vi "AB_820_850_Project_SourceItems.vi"(5 "Provider Item":T1, 7 "action":T3, 8 "error in (no error)":errorcluster, 9 "buildType":T2, 10 "oldBuildObject":T1, 11 "buildObject":T1) -> (0 "error out":errorcluster, 3 "buildObject out":T1, 4 "usedDestinations":i32[](array[numeric]))   [LabVIEW 2020]
doc: "Reads and writes the data to the object property bag."
uses:
  <resource>/Framework/Providers/API/ItemRef.ctl
  <vilib>/AppBuilder/RW_Project/AB_RW_Project_PropBag_ArrayAction.ctl
  <vilib>/AppBuilder/AB_BuildType.ctl
  <vilib>/AppBuilder/RW_Project/AB_RW_Project_Source_Data_for_Previous.ctl
  <vilib>/Utility/lvfile.llb/LVFileType.ctl
  <vilib>/AppBuilder/RW_Project/AB_RW_Project_PropBag_Action.ctl
  <vilib>/AppBuilder/AB_Source_Inclusion.ctl
  <vilib>/Utility/lvfile.llb/NI_FileType.lvlib
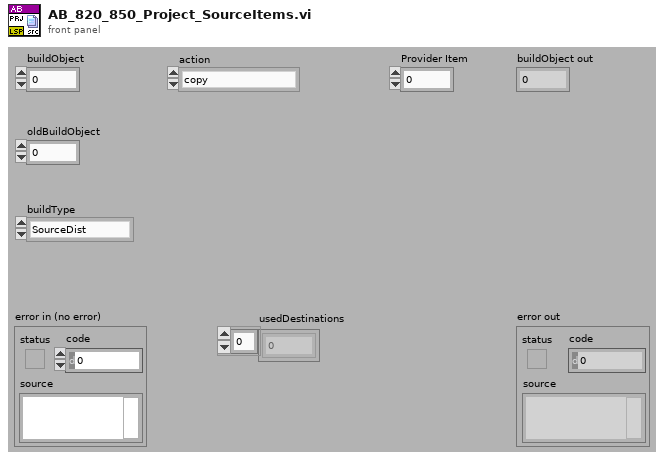
[diagram p1: front panel]
types:
  T1 = typedef "ItemRef.ctl" = u64
  T2 = typedef "AB_BuildType.ctl" = enum16{"SourceDist", "EXE", "DLL", "RTExe"}
  T3 = typedef "AB_RW_Project_PropBag_ArrayAction.ctl" = enum16{"copy", "saveForPrevious", "loadFromPrevious", "clear"}
  T4 = typedef "AB_RW_Project_Source_Data_for_Previous.ctl" = cluster{"buildType":T2, "folder":bool, "linkerInfo":cluster{"path":path, "delimited name":string, "type":T5, "iState":u32, "iStyle":u16, "wStyle":u16, "buttons":u16, "viflags":u32, "viflags2":u32, "links":u32[]}, "isLibrary":bool}
  T5 = typedef "NI_FileType.lvlib/LVFileType.ctl" = enum32{"Invalid file", "Unknown type", "Instrument", "Control", "Polymorphic VI", "Project", "Library", "LVClass", "XControl", "XNode", "Shared library", ".NET assembly", "ActiveX interface", "CIN", "Run-time menu", "Palette menu", "Help file", "LLB", "XNode Edit Dependency", "Class Private Data Control", "Statechart", "MathScript .m file", "Ladder Diagram", "LVLibp", "XNode Build Dependency"}
  T6 = typedef "AB_RW_Project_PropBag_Action.ctl" = enum16{"read", "write", "clear", "readPrevious", "writePrevious", "clearPrevious"}
  T7 = typedef "AB_Source_Inclusion.ctl" = enum16{"IncludeIfReferenced", "Include", "Exclude", "TopLevel"}
  T8 = cluster{"itemID":string, "sourceInclusion":T7, "destinationIndex":i32, "properties":cluster{"sourcePropertyType":enum16{"Remove block diagram", "Remove front panel", "Password", "Window has title bar", "Show menu bar", "Show vertical scroll bar", "Show horizontal scroll bar", "Show toolbar", "Show Abort button", "Show fp when called", "Window behavior", "Allow user to close window", "Window run-time position", "Run when opened", "Allow debugging", "Auto error handling"}, "value":variant}[], "newName":string, "lvfile":bool}
  T9 = cluster{"LLBtopLevel":bool, "privateDataControl":bool}
  T10 = typedef "ABAPI Dist VI Proto Info.ctl" = cluster{"cptm":string, "params":cluster{"name":string, "dir":enum32{"in", "out", "in/out", "length"}, "inputIdx":i32, "outputIdx":i32, "passBy":i32, "lenInput":i32, "lenOutput":i32}[], "callingConv":i32, "name":string}
  T11 = cluster{"applyInclusion":bool, "applyDestination":bool, "applyProperties":bool, "applyPassword":bool, "applyPrefix":bool, "applySaveSetttings":bool}
  T12 = cluster{"relinkCallers":bool, "atomicCopy":bool, "allowMissingMembers":bool}
  T13 = cluster{"Source":cluster{"itemID":string, "sourceInclusion":T7, "destinationIndex":i32, "properties":cluster{"sourcePropertyType":enum16{"Remove block diagram", "Remove front panel", "Password", "Window has title bar", "Show menu bar", "Show vertical scroll bar", "Show horizontal scroll bar", "Show toolbar", "Show Abort button", "Show fp when called", "Window behavior", "Allow user to close window", "Window run-time position", "Run when opened", "Allow debugging", "Auto error handling"}, "value":variant}[], "newName":string, "lvfile":bool}, "Container":cluster{"applyInclusion":bool, "applyDestination":bool, "applyProperties":bool, "applyPassword":bool, "applyPrefix":bool, "applySaveSetttings":bool}}
  T14 = cluster{"path":path, "delimited name":string, "type":T5, "iState":u32, "iStyle":u16, "wStyle":u16, "buttons":u16, "viflags":u32, "viflags2":u32, "links":u32[]}
  T15 = cluster{"dataSource out":cluster{"itemID":string, "sourceInclusion":T7, "destinationIndex":i32, "properties":cluster{"sourcePropertyType":enum16{"Remove block diagram", "Remove front panel", "Password", "Window has title bar", "Show menu bar", "Show vertical scroll bar", "Show horizontal scroll bar", "Show toolbar", "Show Abort button", "Show fp when called", "Window behavior", "Allow user to close window", "Window run-time position", "Run when opened", "Allow debugging", "Auto error handling"}, "value":variant}[], "newName":string, "lvfile":bool}, "dataSource out":cluster{"applyInclusion":bool, "applyDestination":bool, "applyProperties":bool, "applyPassword":bool, "applyPrefix":bool, "applySaveSetttings":bool}}
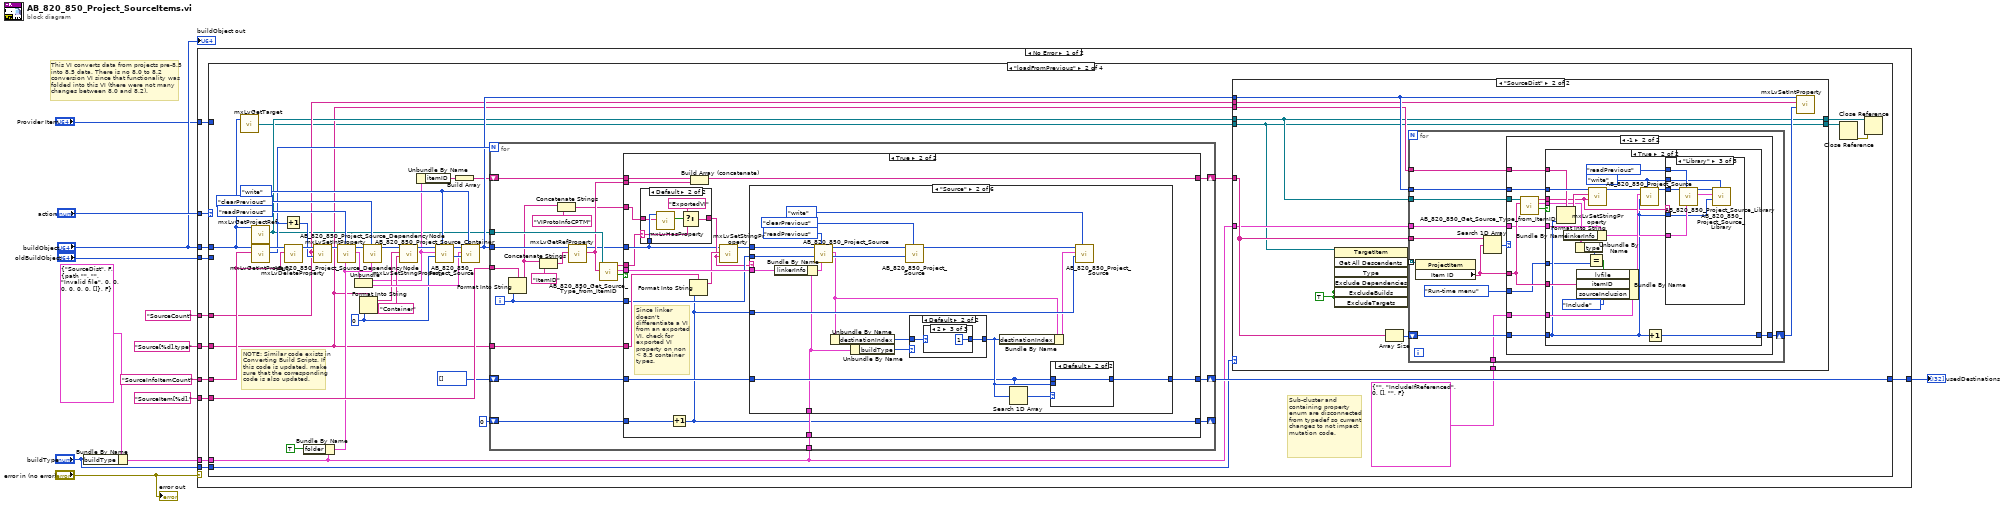
[diagram p0: block diagram]
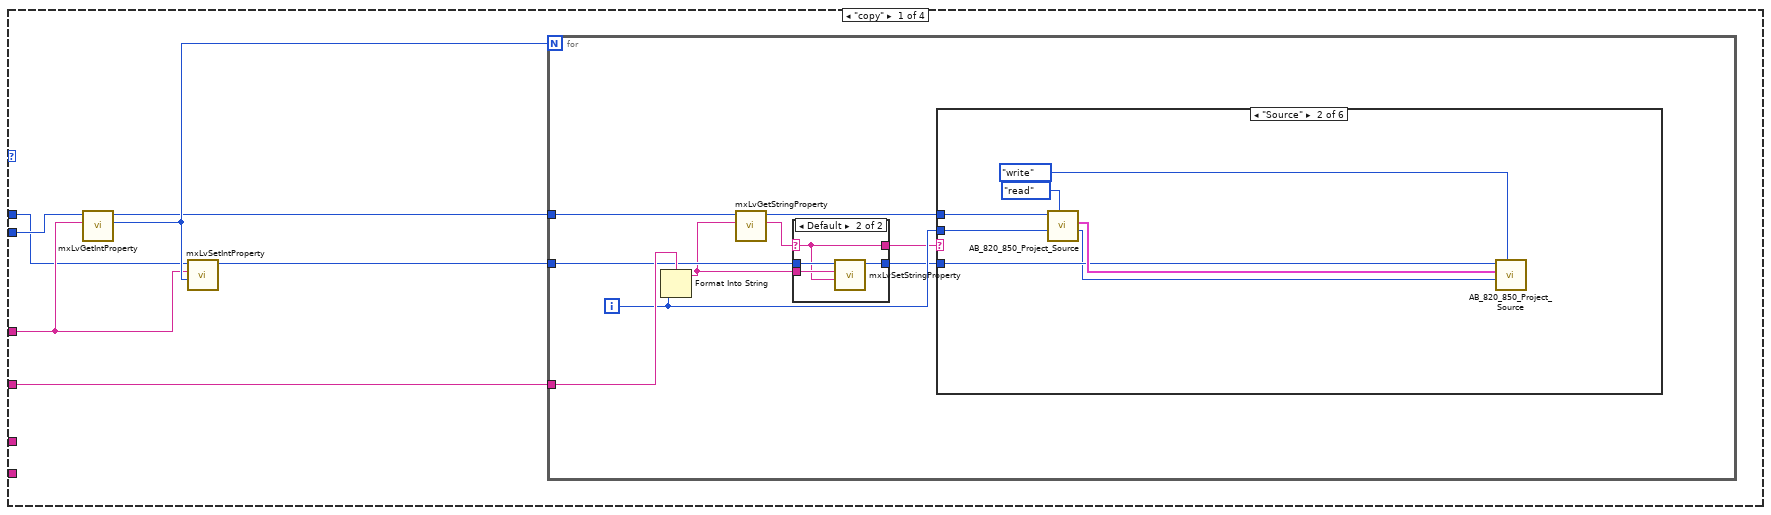
[diagram p2: hidden frame]
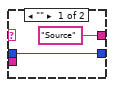
[diagram p3: hidden frame]
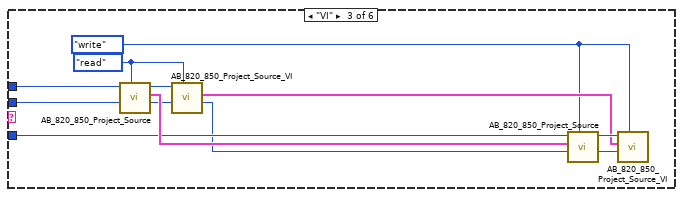
[diagram p5: hidden frame]
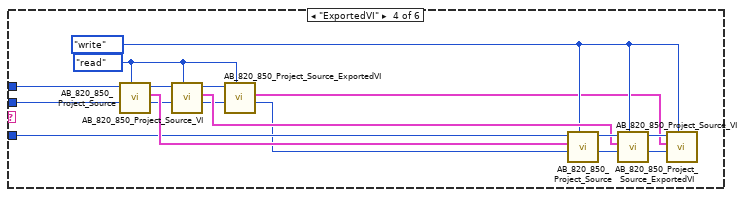
[diagram p6: hidden frame]
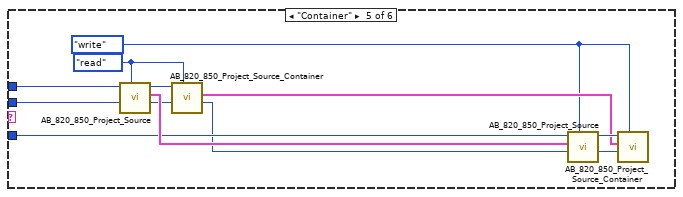
[diagram p7: hidden frame]
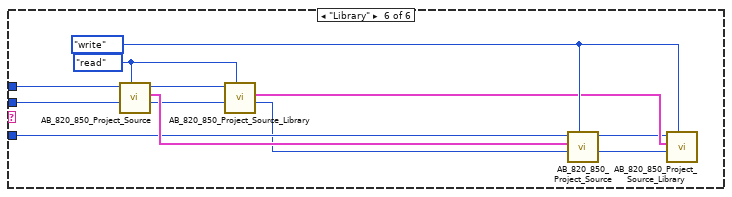
[diagram p8: hidden frame]
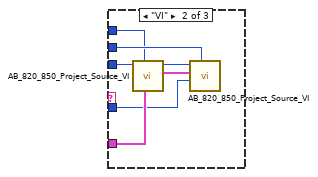
[diagram p13: hidden frame]
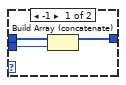
[diagram p17: hidden frame]
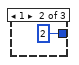
[diagram p20: hidden frame]
diagram:
  # "This VI converts data from projects pre-8.5 into 8.5 data. There is no 8.0 to 8.2 conversion VI since that functionality was folded into this VI (there were not many changes between 8.0 and 8.2)."
  n1 = Bundle By Name(cluster=T4 {"buildType"=enum."SourceDist", "folder"=FALSE, "linkerInfo"={"path"=path "", "delimited name"="", "type"=enum."Invalid file", "iState"=0, "iStyle"=0, "wStyle"=0, "buttons"=0, "viflags"=0, "viflags2"=0, "links"=[]}, "isLibrary"=FALSE} ("dataForPrevious"), "buildType"="buildType") -> (w5:T4)
  n2 = case shown="No Error" "error in (no error)" {
    tunnel: "action" -> [w24 _]
    tunnel: "buildObject" -> [w23 _]
    tunnel: "SourceCount" -> [w22 _]
    tunnel: "Source[%d].type" -> [w21 _]
    tunnel: "SourceInfoItemCount" ("Tag") -> [w20 _]
    tunnel: "SourceItem[%d]." -> [w19 _]
    tunnel: w5 -> [w18 _]
    tunnel: "oldBuildObject" -> [w17 _]
    tunnel: [w16 _] -> w3
    tunnel: "buildType" -> [w15 _]
    tunnel: "Provider Item" -> [w14 _]
    frame No Error {
      n3 = case shown="\"loadFromPrevious\"" w24 {
        tunnel: w23 -> [w25 w123 w454 w723]
        tunnel: w22 -> [w29 w121 w477 w718]
        tunnel: w21 -> [w31 w112 w461 w722]
        tunnel: w20 -> [_ w134 w448 _]
        tunnel: w19 -> [_ w147 _ _]
        tunnel: w18 -> [_ w119 w449 _]
        tunnel: w17 -> [w26 _ _ _]
        tunnel: [_ w129 w464 _] -> w16
        tunnel: w15 -> [_ w120 w452 _]
        tunnel: w14 -> [_ _ w447 _]
        frame "copy" {
          n4 = call <resource>:"mxLvGetIntProperty.vi"("Tag"=w29, "Item"=w26) -> ("Value"=w30:i32, "Item"=w28:T1)  [unwired: 7 in, 1 out]
          n5 = call <resource>:"mxLvSetIntProperty.vi"("Value (0)"=w30, "Tag"=w29, "Item"=w25) -> ("Item"=w27:T1)  [unwired: 7 in, 1 out]
          n6 = for {
            N: w30 -> [_]
            tunnel: w31 -> [w40]
            tunnel: w28 -> [w39]
            tunnel: w27 -> [w37]
            i -> [w38]
            n7 = Format Into String(format string=w40, w38) -> (resulting string=w34:string)  [unwired: 2 in, 1 out]
            n8 = call <resource>:"mxLvGetStringProperty.vi"("Tag"=w34, "Item"=w39) -> ("Value"=w33:string, "Item"=w36:T1)  [unwired: 7 in, 1 out]
            n9 = case shown="Default" w33 {
              selector: w33 -> [_ w43]
              tunnel: w37 -> [w41 w46]
              tunnel: [w41 w45] -> w35
              tunnel: w34 -> [_ w44]
              tunnel: ["Source" w43] -> w32
              frame "" {
              }
              frame Default {
                n10 = call <resource>:"mxLvSetStringProperty.vi"("Value (\"\")"=w43, "Tag"=w44, "Item"=w46) -> ("Item"=w45:T1)  [unwired: 7 in, 1 out]
              }
            }
            n11 = case shown="\"Source\"" w32 {
              tunnel: w36 -> [_ w53 w65 w82 w94 w106]
              tunnel: w38 -> [_ w52 w64 w81 w93 w105]
              tunnel: w35 -> [_ w48 w56 w74 w85 w103]
              frame Default {
              }
              frame "Source" {
                n12 = call <vilib>:"AB_820_850_Project_Source.vi"("action"=AB_RW_Project_PropBag_Action."read", "index in"=w52, "buildObject"=w53) -> ("index out"=w47:i32, "dataSource out"=w49:T8)  [unwired: 5 in, 2 out]
                n13 = call <vilib>:"AB_820_850_Project_Source.vi"("action"=AB_RW_Project_PropBag_Action."write", "index in"=w47, "dataSource in"=w49, "buildObject"=w48) -> ()  [unwired: 4 in, 4 out]
              }
              frame "VI" {
                w54 = AB_RW_Project_PropBag_Action."write" ("action")
                w60 = AB_RW_Project_PropBag_Action."read" ("action")
                n14 = call <vilib>:"AB_820_850_Project_Source.vi"("action"=w60, "index in"=w64, "buildObject"=w65) -> ("index out"=w61:i32, "dataSource out"=w63:T8, "buildObject out"=w62:T1)  [unwired: 5 in, 1 out]
                n15 = call <vilib>:"AB_820_850_Project_Source_VI.vi"("action"=w60, "index in"=w61, "buildObject"=w62) -> ("index out"=w55:i32, "dataSource out"=w57:T9)  [unwired: 5 in, 2 out]
                n16 = call <vilib>:"AB_820_850_Project_Source.vi"("action"=w54, "index in"=w55, "dataSource in"=w63, "buildObject"=w56) -> ("index out"=w58:i32, "buildObject out"=w59:T1)  [unwired: 4 in, 2 out]
                n17 = call <vilib>:"AB_820_850_Project_Source_VI.vi"("action"=w54, "index in"=w58, "dataSource in"=w57, "buildObject"=w59) -> ()  [unwired: 4 in, 4 out]
              }
              frame "ExportedVI" {
                w67 = AB_RW_Project_PropBag_Action."write" ("action")
                w72 = AB_RW_Project_PropBag_Action."read" ("action")
                n18 = call <vilib>:"AB_820_850_Project_Source.vi"("action"=w72, "index in"=w81, "buildObject"=w82) -> ("index out"=w78:i32, "dataSource out"=w80:T8, "buildObject out"=w79:T1)  [unwired: 5 in, 1 out]
                n19 = call <vilib>:"AB_820_850_Project_Source_VI.vi"("action"=w72, "index in"=w78, "buildObject"=w79) -> ("index out"=w71:i32, "dataSource out"=w75:T9, "buildObject out"=w73:T1)  [unwired: 5 in, 1 out]
                n20 = call <vilib>:"AB_820_850_Project_Source_ExportedVI.vi"("action"=w72, "index in"=w71, "buildObject"=w73) -> ("index out"=w70:i32, "dataSource out"=w66:cluster{"vipInfo":T10})  [unwired: 5 in, 2 out]
                n21 = call <vilib>:"AB_820_850_Project_Source.vi"("action"=w67, "index in"=w70, "dataSource in"=w80, "buildObject"=w74) -> ("index out"=w76:i32, "buildObject out"=w77:T1)  [unwired: 4 in, 2 out]
                n22 = call <vilib>:"AB_820_850_Project_Source_VI.vi"("action"=w67, "index in"=w76, "dataSource in"=w75, "buildObject"=w77) -> ("index out"=w68:i32, "buildObject out"=w69:T1)  [unwired: 4 in, 2 out]
                n23 = call <vilib>:"AB_820_850_Project_Source_ExportedVI.vi"("action"=w67, "index in"=w68, "dataSource in"=w66, "buildObject"=w69) -> ()  [unwired: 4 in, 4 out]
              }
              frame "Container" {
                w84 = AB_RW_Project_PropBag_Action."write" ("action")
                w89 = AB_RW_Project_PropBag_Action."read" ("action")
                n24 = call <vilib>:"AB_820_850_Project_Source.vi"("action"=w89, "index in"=w93, "buildObject"=w94) -> ("index out"=w86:i32, "dataSource out"=w92:T8, "buildObject out"=w91:T1)  [unwired: 5 in, 1 out]
                n25 = call <vilib>:"AB_820_850_Project_Source_Container.vi"("action"=w89, "index in"=w86, "buildObject"=w91) -> ("index out"=w83:i32, "dataSource out"=w88:T11)  [unwired: 5 in, 2 out]
                n26 = call <vilib>:"AB_820_850_Project_Source.vi"("action"=w84, "index in"=w83, "dataSource in"=w92, "buildObject"=w85) -> ("index out"=w87:i32, "buildObject out"=w90:T1)  [unwired: 4 in, 2 out]
                n27 = call <vilib>:"AB_820_850_Project_Source_Container.vi"("action"=w84, "index in"=w87, "dataSource in"=w88, "buildObject"=w90) -> ()  [unwired: 4 in, 4 out]
              }
              frame "Library" {
                w101 = AB_RW_Project_PropBag_Action."write" ("action")
                w100 = AB_RW_Project_PropBag_Action."read" ("action")
                n28 = call <vilib>:"AB_820_850_Project_Source.vi"("action"=w100, "index in"=w105, "buildObject"=w106) -> ("index out"=w97:i32, "dataSource out"=w104:T8, "buildObject out"=w98:T1)  [unwired: 5 in, 1 out]
                n29 = call <vilib>:"AB_820_850_Project_Source_Library.vi"("action"=w100, "index in"=w97, "buildObject"=w98) -> ("index out"=w102:i32, "dataSource out"=w99:T12)  [unwired: 5 in, 2 out]
                n30 = call <vilib>:"AB_820_850_Project_Source.vi"("action"=w101, "index in"=w102, "dataSource in"=w104, "buildObject"=w103) -> ("index out"=w95:i32, "buildObject out"=w96:T1)  [unwired: 4 in, 2 out]
                n31 = call <vilib>:"AB_820_850_Project_Source_Library.vi"("action"=w101, "index in"=w95, "dataSource in"=w99, "buildObject"=w96) -> ()  [unwired: 4 in, 4 out]
              }
            }
          }
        }
        frame "loadFromPrevious" {
          w125 = 0 ("index in")
          w138 = AB_RW_Project_PropBag_Action."write" ("action")
          # "Sub-cluster and containing property enum are disconnected from typedef so current changes to not impact mutation code."
          # "NOTE: Similar code exists in Converting Build Scripts. If this code is updated, make sure that the corresponding code is also updated."
          n32 = call <resource>:"mxLvGetTarget.vi"("Item"=w123) -> ("Target"=w110:refnum<vi>)  [unwired: 1 in, 2 out]
          n33 = call <resource>:"mxLvGetProjectRef.vi"("Item"=w123) -> ("Project Refnum"=w113:refnum<vi>)  [unwired: 8 in, 2 out]
          n34 = call <resource>:"mxLvGetIntProperty.vi"("Tag"=w134, "Item"=w123) -> ("Value"=w132:i32, "Item"=w136:T1)  [unwired: 7 in, 1 out]
          n35 = Increment(x=w132) -> (x+1=w131:i32)
          n36 = call <resource>:"mxLvDeleteProperty.vi"("Tag"=w134, "Item"=w136) -> ("Item"=w135:T1)  [unwired: 8 in, 1 out]
          n37 = Bundle By Name(cluster=w119, "folder"=TRUE) -> (w143:T4)
          n38 = call <resource>:"mxLvSetIntProperty.vi"("Value (0)"=w131, "Tag"=w121, "Item"=w135) -> ("Item"=w133:T1)  [unwired: 7 in, 1 out]
          n39 = call <vilib>:"AB_820_850_Project_Source_DependencyNode.vi"("dataForPrevious"=w143, "action"=AB_RW_Project_PropBag_Action."readPrevious", "buildObject in"=w133) -> ("data out"=w141:T13, "buildObject out"=w145:T1)  [unwired: 6 in, 1 out]
          n40 = Unbundle(w141) -> ("Source"=w117:T8, "Container"=w137:T11)
          n41 = Format Into String(format string=w112, w125) -> (resulting string=w124:string)  [unwired: 2 in, 1 out]
          n42 = call <vilib>:"AB_820_850_Project_Source_DependencyNode.vi"("dataForPrevious"=w143, "action"=AB_RW_Project_PropBag_Action."clearPrevious", "buildObject in"=w145) -> ("buildObject out"=w128:T1)  [unwired: 6 in, 2 out]
          n43 = call <resource>:"mxLvSetStringProperty.vi"("Value (\"\")"="Container", "Tag"=w124, "Item"=w128) -> ("Item"=w127:T1)  [unwired: 7 in, 1 out]
          n44 = Unbundle By Name(w117) -> ("itemID"=w118:string)
          n45 = call <vilib>:"AB_820_850_Project_Source.vi"("action"=w138, "index in"=w125, "dataSource in"=w117, "buildObject"=w127) -> ("index out"=w139:i32, "buildObject out"=w140:T1)  [unwired: 4 in, 2 out]
          n46 = Build Array(w118) -> (w116:string[])
          n47 = call <vilib>:"AB_820_850_Project_Source_Container.vi"("action"=w138, "index in"=w139, "dataSource in"=w137, "buildObject"=w140) -> ("buildObject out"=w122:T1)  [unwired: 4 in, 3 out]
          n48 = for {
            N: w132 -> [_]
            tunnel: w122 -> [w240]
            tunnel: w147 -> [w243]
            tunnel: w113 -> [w239]
            tunnel: w119 -> [w237]
            tunnel: w112 -> [w236]
            shift-right: [w234] -> w129
            shift-left: i32[] [] -> [w233]
            shift-right: [w228] -> w115
            shift-left: w116 -> [w229]
            shift-right: [w224] -> _
            shift-left: 0 -> [w225]
            i -> [w235]
            n49 = Format Into String(format string=w243, w235) -> (resulting string=w231:string)  [unwired: 2 in, 1 out]
            n50 = Concatenate Strings(w231, "ItemID") -> (w241:string)
            n51 = Concatenate Strings(w231, "VIProtoInfoCPTM") -> (w223:string)
            n52 = call <resource>:"mxLvGetRefProperty.vi"("Tag"=w241, "Item"=w240) -> ("Value"=w227:string, "Item"=w222:T1)  [unwired: 7 in, 1 out]
            n53 = call <vilib>:"AB_820_850_Get_Source_Type_from_ItemID.vi"("Item ID"=w227, "Project Refnum"=w239) -> ("valid?"=w226:bool, "linkerInfo"=w238:T14, "classType"=w230:string)  [unwired: 6 in, 1 out]
            n54 = case shown="True" w226 {
              tunnel: w238 -> [_ w263]
              tunnel: w237 -> [_ w262]
              tunnel: w236 -> [_ w260]
              tunnel: w235 -> [_ w259]
              tunnel: [w245 w257] -> w234
              tunnel: w233 -> [w245 w256]
              tunnel: w230 -> [_ w247]
              tunnel: w229 -> [w246 w254]
              tunnel: [w246 w253] -> w228
              tunnel: w227 -> [_ w252]
              tunnel: w225 -> [w244 w251]
              tunnel: [w244 w250] -> w224
              tunnel: w223 -> [_ w248]
              tunnel: w222 -> [_ w249]
              frame False {
              }
              frame True {
                # "Since linker doesn't differentiate a VI from an exported VI, check for exported VI property on non  < 8.5 container types."
                n55 = case shown="Default" w247 {
                  selector: w247 -> [w264 w265]
                  tunnel: [w264 w270] -> w255
                  tunnel: w249 -> [_ w268]
                  tunnel: w248 -> [_ w267]
                  frame "Container", "Library" {
                  }
                  frame Default {
                    n56 = call <resource>:"mxLvHasProperty.vi"("Tag"=w267, "Item"=w268) -> ("HasProperty"=w266:bool)  [unwired: 7 in, 2 out]
                    n57 = Select(t="ExportedVI", s=w266, f=w265) -> (s? t:f=w270:string)
                  }
                }
                n58 = Increment(x=w251) -> (x+1=w250:i32)
                n59 = Format Into String(format string=w260, w250) -> (resulting string=w258:string)  [unwired: 2 in, 1 out]
                n60 = Build Array (concatenate)(w254, w252) -> (w253:string[])
                n61 = call <resource>:"mxLvSetStringProperty.vi"("Value (\"\")"=w255, "Tag"=w258, "Item"=w249) -> ("Item"=w261:T1)  [unwired: 7 in, 1 out]
                n62 = case shown="\"Source\"" w255 {
                  tunnel: w263 -> [_ w272 w322 w366 _ w432]
                  tunnel: w261 -> [_ w291 w326 w368 w401 w436]
                  tunnel: w259 -> [_ w290 w325 w367 w400 w435]
                  tunnel: w262 -> [_ w274 w311 w359 w379 w418]
                  tunnel: w250 -> [_ w283 w312 w360 w397 w431]
                  tunnel: [w271 w278 w304 w352 w383 w421] -> w257
                  tunnel: w256 -> [w271 w275 w303 w351 w380 w417]
                  frame Default {
                  }
                  frame "Source" {
                    n63 = Bundle By Name(cluster=w274, "linkerInfo"=w272) -> (w273:T4)
                    n64 = call <vilib>:"AB_820_850_Project_Source.vi"("dataForPrevious"=w273, "action"=AB_RW_Project_PropBag_Action."readPrevious", "index in"=w290, "buildObject"=w291) -> ("index out"=w284:i32, "dataSource out"=w277:T8, "buildObject out"=w286:T1)  [unwired: 4 in, 1 out]
                    n65 = Unbundle By Name(w277) -> ("destinationIndex"=w281:i32)
                    n66 = Unbundle By Name(w274) -> ("buildType"=w282:T2)
                    n67 = call <vilib>:"AB_820_850_Project_Source.vi"("action"=AB_RW_Project_PropBag_Action."clearPrevious", "index in"=w284, "buildObject"=w286) -> ("buildObject out"=w285:T1)  [unwired: 5 in, 3 out]
                    n68 = case shown="Default" w282 {
                      tunnel: w281 -> [w296 w298]
                      tunnel: [w296 w297] -> w279
                      frame "SourceDist" {
                      }
                      frame Default {
                        n69 = case shown="2" w298 {
                          selector: w298 -> [w299 _ _]
                          tunnel: [w299 2 ("destinationIndex") 1 ("destinationIndex")] -> w297
                          frame Default {
                          }
                          frame 1 {
                          }
                          frame 2 {
                          }
                        }
                      }
                    }
                    n70 = Bundle By Name(cluster=w277, "destinationIndex"=w279) -> (w276:T8)
                    n71 = Search 1D Array(1D array=w275, element=w279) -> (index of element=w280:i32)  [unwired: 1 in]
                    n72 = case shown="Default" w280 {
                      tunnel: w279 -> [w294 _]
                      tunnel: [w293 w295] -> w278
                      tunnel: w275 -> [w292 w295]
                      frame -1 {
                        n73 = Build Array (concatenate)(w292, w294) -> (w293:i32[])
                      }
                      frame Default {
                      }
                    }
                    n74 = call <vilib>:"AB_820_850_Project_Source.vi"("action"=AB_RW_Project_PropBag_Action."write", "index in"=w283, "dataSource in"=w276, "buildObject"=w285) -> ()  [unwired: 4 in, 4 out]
                  }
                  frame "VI" {
                    w316 = AB_RW_Project_PropBag_Action."write" ("action")
                    w317 = AB_RW_Project_PropBag_Action."readPrevious" ("action")
                    n75 = Bundle By Name(cluster=w311, "linkerInfo"=w322) -> (w302:T4)
                    n76 = call <vilib>:"AB_820_850_Project_Source.vi"("dataForPrevious"=w302, "action"=w317, "index in"=w325, "buildObject"=w326) -> ("index out"=w320:i32, "dataSource out"=w308:T8, "buildObject out"=w321:T1)  [unwired: 4 in, 1 out]
                    n77 = Unbundle By Name(w308) -> ("destinationIndex"=w309:i32)
                    n78 = call <vilib>:"AB_820_850_Project_Source_VI.vi"("dataForPrevious"=w302, "action"=w317, "index in"=w320, "buildObject"=w321) -> ("index out"=w319:i32, "dataSource out"=w313:T9, "buildObject out"=w318:T1)  [unwired: 4 in, 1 out]
                    n79 = Unbundle By Name(w311) -> ("buildType"=w310:T2)
                    n80 = call <vilib>:"AB_820_850_Project_Source.vi"("action"=AB_RW_Project_PropBag_Action."clearPrevious", "index in"=w319, "buildObject"=w318) -> ("buildObject out"=w323:T1)  [unwired: 5 in, 3 out]
                    n81 = case shown="Default" w310 {
                      tunnel: w309 -> [w331 w333]
                      tunnel: [w331 w332] -> w305
                      frame "SourceDist" {
                      }
                      frame Default {
                        n82 = case shown="2" w333 {
                          selector: w333 -> [w334 _ _]
                          tunnel: [w334 2 ("destinationIndex") 1 ("destinationIndex")] -> w332
                          frame Default {
                          }
                          frame 1 {
                          }
                          frame 2 {
                          }
                        }
                      }
                    }
                    n83 = Bundle By Name(cluster=w308, "destinationIndex"=w305) -> (w307:T8)
                    n84 = Search 1D Array(1D array=w303, element=w305) -> (index of element=w306:i32)  [unwired: 1 in]
                    n85 = case shown="Default" w306 {
                      tunnel: w305 -> [w329 _]
                      tunnel: [w328 w330] -> w304
                      tunnel: w303 -> [w327 w330]
                      frame -1 {
                        n86 = Build Array (concatenate)(w327, w329) -> (w328:i32[])
                      }
                      frame Default {
                      }
                    }
                    n87 = call <vilib>:"AB_820_850_Project_Source.vi"("action"=w316, "index in"=w312, "dataSource in"=w307, "buildObject"=w323) -> ("index out"=w314:i32, "buildObject out"=w315:T1)  [unwired: 4 in, 2 out]
                    n88 = call <vilib>:"AB_820_850_Project_Source_VI.vi"("action"=w316, "index in"=w314, "dataSource in"=w313, "buildObject"=w315) -> ()  [unwired: 4 in, 4 out]
                  }
                  frame "ExportedVI" {
                    w343 = AB_RW_Project_PropBag_Action."write" ("action")
                    w340 = AB_RW_Project_PropBag_Action."clearPrevious" ("action")
                    w346 = AB_RW_Project_PropBag_Action."readPrevious" ("action")
                    n89 = Bundle By Name(cluster=w359, "linkerInfo"=w366) -> (w337:T4)
                    n90 = call <vilib>:"AB_820_850_Project_Source.vi"("dataForPrevious"=w337, "action"=w346, "index in"=w367, "buildObject"=w368) -> ("index out"=w364:i32, "dataSource out"=w356:T8, "buildObject out"=w365:T1)  [unwired: 4 in, 1 out]
                    n91 = Unbundle By Name(w356) -> ("destinationIndex"=w357:i32)
                    n92 = call <vilib>:"AB_820_850_Project_Source_VI.vi"("dataForPrevious"=w337, "action"=w346, "index in"=w364, "buildObject"=w365) -> ("index out"=w348:i32, "dataSource out"=w361:T9, "buildObject out"=w350:T1)  [unwired: 4 in, 1 out]
                    n93 = Unbundle By Name(w359) -> ("buildType"=w358:T2)
                    n94 = call <vilib>:"AB_820_850_Project_Source_ExportedVI.vi"("action"=w346, "index in"=w348, "buildObject"=w350) -> ("index out"=w347:i32, "dataSource out"=w339:cluster{"vipInfo":T10}, "buildObject out"=w349:T1)  [unwired: 5 in, 1 out]
                    n95 = call <vilib>:"AB_820_850_Project_Source.vi"("action"=w340, "index in"=w347, "buildObject"=w349) -> ("index out"=w341:i32, "buildObject out"=w342:T1)  [unwired: 5 in, 2 out]
                    n96 = case shown="Default" w358 {
                      tunnel: w357 -> [w373 w375]
                      tunnel: [w373 w374] -> w353
                      frame "SourceDist" {
                      }
                      frame Default {
                        n97 = case shown="2" w375 {
                          selector: w375 -> [w376 _ _]
                          tunnel: [w376 2 ("destinationIndex") 1 ("destinationIndex")] -> w374
                          frame Default {
                          }
                          frame 1 {
                          }
                          frame 2 {
                          }
                        }
                      }
                    }
                    n98 = call <vilib>:"AB_820_850_Project_Source_ExportedVI.vi"("action"=w340, "index in"=w341, "dataSource in"=w339, "buildObject"=w342) -> ("buildObject out"=w338:T1)  [unwired: 4 in, 3 out]
                    n99 = Bundle By Name(cluster=w356, "destinationIndex"=w353) -> (w355:T8)
                    n100 = Search 1D Array(1D array=w351, element=w353) -> (index of element=w354:i32)  [unwired: 1 in]
                    n101 = case shown="Default" w354 {
                      tunnel: w353 -> [w371 _]
                      tunnel: [w370 w372] -> w352
                      tunnel: w351 -> [w369 w372]
                      frame -1 {
                        n102 = Build Array (concatenate)(w369, w371) -> (w370:i32[])
                      }
                      frame Default {
                      }
                    }
                    n103 = call <vilib>:"AB_820_850_Project_Source.vi"("action"=w343, "index in"=w360, "dataSource in"=w355, "buildObject"=w338) -> ("index out"=w362:i32, "buildObject out"=w363:T1)  [unwired: 4 in, 2 out]
                    n104 = call <vilib>:"AB_820_850_Project_Source_VI.vi"("action"=w343, "index in"=w362, "dataSource in"=w361, "buildObject"=w363) -> ("index out"=w344:i32, "buildObject out"=w345:T1)  [unwired: 4 in, 2 out]
                    n105 = call <vilib>:"AB_820_850_Project_Source_ExportedVI.vi"("action"=w343, "index in"=w344, "dataSource in"=w339, "buildObject"=w345) -> ()  [unwired: 4 in, 4 out]
                  }
                  frame "Container" {
                    w392 = AB_RW_Project_PropBag_Action."write" ("action")
                    w393 = AB_RW_Project_PropBag_Action."readPrevious" ("action")
                    n106 = call <vilib>:"AB_820_850_Project_Source.vi"("dataForPrevious"=w379, "action"=w393, "index in"=w400, "buildObject"=w401) -> ("index out"=w388:i32, "dataSource out"=w382:T8, "buildObject out"=w396:T1)  [unwired: 4 in, 1 out]
                    n107 = Unbundle By Name(w382) -> ("destinationIndex"=w386:i32)
                    n108 = call <vilib>:"AB_820_850_Project_Source_Container.vi"("action"=w393, "index in"=w388, "buildObject"=w396) -> ("index out"=w390:i32, "dataSource out"=w391:T11, "buildObject out"=w395:T1)  [unwired: 5 in, 1 out]
                    n109 = Unbundle By Name(w379) -> ("buildType"=w387:T2)
                    n110 = call <vilib>:"AB_820_850_Project_Source.vi"("action"=AB_RW_Project_PropBag_Action."clearPrevious", "index in"=w390, "buildObject"=w395) -> ("buildObject out"=w398:T1)  [unwired: 5 in, 3 out]
                    n111 = case shown="Default" w387 {
                      tunnel: w386 -> [w406 w408]
                      tunnel: [w406 w407] -> w384
                      frame "SourceDist" {
                      }
                      frame Default {
                        n112 = case shown="2" w408 {
                          selector: w408 -> [w409 _ _]
                          tunnel: [w409 2 ("destinationIndex") 1 ("destinationIndex")] -> w407
                          frame Default {
                          }
                          frame 1 {
                          }
                          frame 2 {
                          }
                        }
                      }
                    }
                    n113 = Bundle By Name(cluster=w382, "destinationIndex"=w384) -> (w381:T8)
                    n114 = Search 1D Array(1D array=w380, element=w384) -> (index of element=w385:i32)  [unwired: 1 in]
                    n115 = case shown="Default" w385 {
                      tunnel: w384 -> [w404 _]
                      tunnel: [w403 w405] -> w383
                      tunnel: w380 -> [w402 w405]
                      frame -1 {
                        n116 = Build Array (concatenate)(w402, w404) -> (w403:i32[])
                      }
                      frame Default {
                      }
                    }
                    n117 = call <vilib>:"AB_820_850_Project_Source.vi"("action"=w392, "index in"=w397, "dataSource in"=w381, "buildObject"=w398) -> ("index out"=w389:i32, "buildObject out"=w394:T1)  [unwired: 4 in, 2 out]
                    n118 = call <vilib>:"AB_820_850_Project_Source_Container.vi"("action"=w392, "index in"=w389, "dataSource in"=w391, "buildObject"=w394) -> ()  [unwired: 4 in, 4 out]
                  }
                  frame "Library" {
                    w426 = AB_RW_Project_PropBag_Action."write" ("action")
                    w428 = AB_RW_Project_PropBag_Action."readPrevious" ("action")
                    n119 = Bundle By Name(cluster=w418, "linkerInfo"=w432) -> (w412:T4)
                    n120 = call <vilib>:"AB_820_850_Project_Source.vi"("dataForPrevious"=w412, "action"=w428, "index in"=w435, "buildObject"=w436) -> ("index out"=w415:i32, "dataSource out"=w419:T8, "buildObject out"=w416:T1)  [unwired: 4 in, 1 out]
                    n121 = Unbundle By Name(w419) -> ("destinationIndex"=w424:i32)
                    n122 = Unbundle By Name(w418) -> ("buildType"=w425:T2)
                    n123 = call <vilib>:"AB_820_850_Project_Source_Library.vi"("dataForPrevious"=w412, "action"=w428, "index in"=w415, "buildObject"=w416) -> ("index out"=w429:i32, "dataSource out"=w427:T12, "buildObject out"=w430:T1)  [unwired: 4 in, 1 out]
                    n124 = call <vilib>:"AB_820_850_Project_Source.vi"("action"=AB_RW_Project_PropBag_Action."clearPrevious", "index in"=w429, "buildObject"=w430) -> ("buildObject out"=w433:T1)  [unwired: 5 in, 3 out]
                    n125 = case shown="Default" w425 {
                      tunnel: w424 -> [w441 w443]
                      tunnel: [w441 w442] -> w422
                      frame "SourceDist" {
                      }
                      frame Default {
                        n126 = case shown="Default" w443 {
                          selector: w443 -> [w444 _ _]
                          tunnel: [w444 2 ("destinationIndex") 1 ("destinationIndex")] -> w442
                          frame Default {
                          }
                          frame 1 {
                          }
                          frame 2 {
                          }
                        }
                      }
                    }
                    n127 = Bundle By Name(cluster=w419, "destinationIndex"=w422) -> (w420:T8)
                    n128 = Search 1D Array(1D array=w417, element=w422) -> (index of element=w423:i32)  [unwired: 1 in]
                    n129 = case shown="Default" w423 {
                      tunnel: w422 -> [w439 _]
                      tunnel: [w438 w440] -> w421
                      tunnel: w417 -> [w437 w440]
                      frame -1 {
                        n130 = Build Array (concatenate)(w437, w439) -> (w438:i32[])
                      }
                      frame Default {
                      }
                    }
                    n131 = call <vilib>:"AB_820_850_Project_Source.vi"("action"=w426, "index in"=w431, "dataSource in"=w420, "buildObject"=w433) -> ("index out"=w414:i32, "buildObject out"=w413:T1)  [unwired: 4 in, 2 out]
                    n132 = call <vilib>:"AB_820_850_Project_Source_Library.vi"("action"=w426, "index in"=w414, "dataSource in"=w427, "buildObject"=w413) -> ()  [unwired: 4 in, 4 out]
                  }
                }
              }
            }
          }
          n133 = case shown="\"SourceDist\"" w120 {
            tunnel: w110 -> [w148 w150]
            tunnel: w115 -> [_ w160]
            tunnel: w122 -> [_ w155]
            tunnel: T8 {"itemID"="", "sourceInclusion"=enum."IncludeIfReferenced", "destinationIndex"=0, "properties"=[], "newName"="", "lvfile"=FALSE} ("dataSource in") -> [_ w158]
            tunnel: w119 -> [_ w157]
            tunnel: w121 -> [_ w154]
            tunnel: w113 -> [w149 w151]
            tunnel: w112 -> [_ w152]
            tunnel: [w149 w151] -> w108
            tunnel: [w148 w150] -> w109
            frame Default {
            }
            frame "SourceDist" {
              w156 = TRUE ("ExcludeDependencies")
              n134 = invoke class="TargetItem" method="Get All Descendents"(reference=w150, "Exclude Dependencies"=w156, "ExcludeBuilds"=w156, "ExcludeTargets"=w156) -> ("All Descendents"=w161:refnum<vi>[])  [unwired: 3 in, 6 out]
              n135 = Array Size(array=w160) -> (size(s)=w159:i32)
              n136 = for {
                tunnel: w161 -> [w173] mode=indexing
                tunnel: w160 -> [w172]
                shift-right: [w168] -> w153
                shift-left: w159 -> [w169]
                tunnel: w155 -> [w171]
                tunnel: w158 -> [w167]
                tunnel: w157 -> [w165]
                tunnel: w151 -> [w164]
                tunnel: w152 -> [w163]
                n137 = property class="ProjectItem"(reference=w173) -> ("Item ID"=w166:string)  [unwired: 1 in, 2 out]
                n138 = Search 1D Array(1D array=w172, element=w166) -> (index of element=w170:i32)  [unwired: 1 in]
                n139 = case shown="-1" w170 {
                  tunnel: w171 -> [_ w184]
                  tunnel: w169 -> [w174 w177]
                  tunnel: [w174 w186] -> w168
                  tunnel: w167 -> [_ w185]
                  tunnel: w166 -> [_ w183]
                  tunnel: w165 -> [_ w179]
                  tunnel: w164 -> [_ w182]
                  tunnel: w163 -> [_ w181]
                  tunnel: LVFileType."Run-time menu" ("x") -> [_ w175]
                  frame Default {
                  }
                  frame -1 {
                    n140 = call <vilib>:"AB_820_850_Get_Source_Type_from_ItemID.vi"("Item ID"=w183, "Project Refnum"=w182) -> ("valid?"=w176:bool, "linkerInfo"=w178:T14, "classType"=w180:string)  [unwired: 6 in, 1 out]
                    n141 = case shown="True" w176 {
                      tunnel: [w187 w207] -> w186
                      tunnel: w185 -> [_ w206]
                      tunnel: w184 -> [_ w203]
                      tunnel: w183 -> [_ w201]
                      tunnel: w181 -> [_ w199]
                      tunnel: w180 -> [_ w198]
                      tunnel: w179 -> [_ w196]
                      tunnel: w178 -> [_ w191]
                      tunnel: w177 -> [w187 w193]
                      tunnel: w175 -> [_ w188]
                      frame False {
                      }
                      frame True {
                        w197 = AB_RW_Project_PropBag_Action."write" ("action")
                        n142 = Format Into String(format string=w199, w193) -> (resulting string=w200:string)  [unwired: 2 in, 1 out]
                        n143 = Bundle By Name(cluster=w196, "linkerInfo"=w191) -> (w195:T4)
                        n144 = Unbundle By Name(w191) -> ("type"=w190:T5)
                        n145 = Equal?(x=w190, y=w188) -> (x = y?=w189:bool)
                        n146 = Bundle By Name(cluster=w206, "lvfile"=w189, "itemID"=w201, "sourceInclusion"=AB_Source_Inclusion."Include") -> (w204:T8)
                        n147 = call <resource>:"mxLvSetStringProperty.vi"("Value (\"\")"=w198, "Tag"=w200, "Item"=w203) -> ("Item"=w202:T1)  [unwired: 7 in, 1 out]
                        n148 = call <vilib>:"AB_820_850_Project_Source.vi"("action"=w197, "index in"=w193, "dataSource in"=w204, "buildObject"=w202) -> ("buildObject out"=w194:T1)  [unwired: 4 in, 3 out]
                        n149 = Increment(x=w193) -> (x+1=w207:i32)
                        n150 = case shown="\"Library\"" w198 {
                          tunnel: w197 -> [_ w210 w217]
                          tunnel: w195 -> [_ w213 w219]
                          tunnel: w194 -> [_ w214 w221]
                          tunnel: w193 -> [_ w209 w215]
                          tunnel: AB_RW_Project_PropBag_Action."readPrevious" ("action") -> [_ w208 w220]
                          frame Default {
                          }
                          frame "VI" {
                            n151 = call <vilib>:"AB_820_850_Project_Source_VI.vi"("dataForPrevious"=w213, "action"=w208, "buildObject"=w214) -> ("dataSource out"=w212:T9, "buildObject out"=w211:T1)  [unwired: 5 in, 2 out]
                            n152 = call <vilib>:"AB_820_850_Project_Source_VI.vi"("action"=w210, "index in"=w209, "dataSource in"=w212, "buildObject"=w211) -> ()  [unwired: 4 in, 4 out]
                          }
                          frame "Library" {
                            n153 = call <vilib>:"AB_820_850_Project_Source_Library.vi"("dataForPrevious"=w219, "action"=w220, "buildObject"=w221) -> ("dataSource out"=w216:T12, "buildObject out"=w218:T1)  [unwired: 5 in, 2 out]
                            n154 = call <vilib>:"AB_820_850_Project_Source_Library.vi"("action"=w217, "index in"=w215, "dataSource in"=w216, "buildObject"=w218) -> ()  [unwired: 4 in, 4 out]
                          }
                        }
                      }
                    }
                  }
                }
              }
              n155 = call <resource>:"mxLvSetIntProperty.vi"("Value (0)"=w153, "Tag"=w154, "Item"=w155) -> ()  [unwired: 7 in, 2 out]
            }
          }
          n156 = Close Reference(reference=w109) -> (error out=w107:errorcluster)  [unwired: 1 in]
          n157 = Close Reference(reference=w108, error in (no error)=w107) -> ()  [unwired: 1 out]
        }
        frame "saveForPrevious" {
          w470 = AB_RW_Project_PropBag_Action."clear" ("action")
          w475 = AB_RW_Project_PropBag_Action."read" ("action")
          # "Sub-cluster and containing property enum are disconnected from typedef so current changes to not impact mutation code."
          # "Dependency node"
          n158 = call <resource>:"mxLvGetIntProperty.vi"("Tag"=w477, "Item"=w454) -> ("Value"=w458:i32, "Item"=w479:T1)  [unwired: 7 in, 1 out]
          n159 = Decrement(x=w458) -> (x-1=w476:i32)
          n160 = call <resource>:"mxLvDeleteProperty.vi"("Tag"=w477, "Item"=w479) -> ("Item"=w478:T1)  [unwired: 8 in, 1 out]
          n161 = Bundle By Name(cluster=w449, "folder"=TRUE) -> (w484:T4)
          n162 = call <resource>:"mxLvSetIntProperty.vi"("Value (0)"=w476, "Tag"=w448, "Item"=w478) -> ("Item"=w474:T1)  [unwired: 7 in, 1 out]
          n163 = call <vilib>:"AB_820_850_Project_Source.vi"("action"=w475, "index in"=0, "buildObject"=w474) -> ("index out"=w480:i32, "dataSource out"=w457:T8, "buildObject out"=w482:T1)  [unwired: 5 in, 1 out]
          n164 = Unbundle By Name(w457) -> ("itemID"=w456:string)
          n165 = call <vilib>:"AB_820_850_Project_Source_Container.vi"("action"=w475, "index in"=w480, "buildObject"=w482) -> ("index out"=w469:i32, "dataSource out"=w473:T11, "buildObject out"=w472:T1)  [unwired: 5 in, 1 out]
          n166 = Build Array(w456) -> (w455:string[])
          n167 = Bundle("dataSource out"=w457, "dataSource out"=w473) -> (w465:T15)  [unwired: 1 in]
          n168 = call <vilib>:"AB_820_850_Project_Source.vi"("action"=w470, "index in"=w469, "buildObject"=w472) -> ("index out"=w468:i32, "buildObject out"=w471:T1)  [unwired: 5 in, 2 out]
          n169 = call <vilib>:"AB_820_850_Project_Source_Container.vi"("action"=w470, "index in"=w468, "buildObject"=w471) -> ("buildObject out"=w467:T1)  [unwired: 5 in, 3 out]
          n170 = Format Into String(format string=w461, 0 ("input 1")) -> (resulting string=w460:string)  [unwired: 2 in, 1 out]
          n171 = call <vilib>:"AB_820_850_Project_Source_DependencyNode.vi"("dataForPrevious"=w484, "action"=AB_RW_Project_PropBag_Action."writePrevious", "data in"=w465, "buildObject in"=w467) -> ("buildObject out"=w462:T1)  [unwired: 5 in, 2 out]
          n172 = call <resource>:"mxLvDeleteProperty.vi"("Tag"=w460, "Item"=w462) -> ("Item"=w451:T1)  [unwired: 8 in, 1 out]
          n173 = for {
            N: w476 -> [_]
            tunnel: w449 -> [w527]
            tunnel: w461 -> [w526]
            tunnel: w451 -> [w525]
            shift-right: [w518] -> w464
            shift-left: i32[] [] -> [w517]
            shift-right: [w515] -> w453
            shift-left: w455 -> [w514]
            i -> [w520]
            n174 = Increment(x=w520) -> (x+1=w521:i32)
            n175 = Format Into String(format string=w526, w521) -> (resulting string=w519:string)  [unwired: 2 in, 1 out]
            n176 = call <resource>:"mxLvGetStringProperty.vi"("Tag"=w519, "Item"=w525) -> ("Value"=w523:string, "Item"=w524:T1)  [unwired: 7 in, 1 out]
            n177 = call <resource>:"mxLvDeleteProperty.vi"("Tag"=w519, "Item"=w524) -> ("Item"=w522:T1)  [unwired: 8 in, 1 out]
            n178 = case shown="\"VI\"" w523 {
              tunnel: w522 -> [_ w548 w584 w595 w669 w707]
              tunnel: w521 -> [_ w547 w583 w631 w668 w706]
              tunnel: w527 -> [_ w532 w561 w615 w644 w691]
              tunnel: w520 -> [_ w540 w573 w625 w667 w705]
              tunnel: [w529 w535 w564 w618 w647 w692] -> w518
              tunnel: w517 -> [w529 w531 w560 w614 w643 w688]
              tunnel: ["" w530 w559 w601 w642 w681] -> w516
              frame Default {
              }
              frame "Source" {
                n179 = call <vilib>:"AB_820_850_Project_Source.vi"("action"=AB_RW_Project_PropBag_Action."read", "index in"=w547, "buildObject"=w548) -> ("index out"=w541:i32, "dataSource out"=w533:T8, "buildObject out"=w543:T1)  [unwired: 5 in, 1 out]
                n180 = Unbundle By Name(w533) -> ("itemID"=w530:string, "destinationIndex"=w538:i32)
                n181 = Unbundle By Name(w532) -> ("buildType"=w539:T2)
                n182 = call <vilib>:"AB_820_850_Project_Source.vi"("action"=AB_RW_Project_PropBag_Action."clear", "index in"=w541, "buildObject"=w543) -> ("buildObject out"=w542:T1)  [unwired: 5 in, 3 out]
                n183 = case shown="\"SourceDist\"" w539 {
                  tunnel: w538 -> [w553 w555]
                  tunnel: [w553 w554] -> w536
                  frame "SourceDist" {
                  }
                  frame Default {
                    n184 = case shown="2" w555 {
                      selector: w555 -> [w556 _ _]
                      tunnel: [w556 2 ("destinationIndex") 1 ("destinationIndex")] -> w554
                      frame Default {
                      }
                      frame 1 {
                      }
                      frame 2 {
                      }
                    }
                  }
                }
                n185 = Bundle By Name(cluster=w533, "destinationIndex"=w536) -> (w534:T8)
                n186 = Search 1D Array(1D array=w531, element=w536) -> (index of element=w537:i32)  [unwired: 1 in]
                n187 = case shown="Default" w537 {
                  tunnel: w536 -> [w551 _]
                  tunnel: [w550 w552] -> w535
                  tunnel: w531 -> [w549 w552]
                  frame -1 {
                    n188 = Build Array (concatenate)(w549, w551) -> (w550:i32[])
                  }
                  frame Default {
                  }
                }
                n189 = call <vilib>:"AB_820_850_Project_Source.vi"("dataForPrevious"=w532, "action"=AB_RW_Project_PropBag_Action."writePrevious", "index in"=w540, "dataSource in"=w534, "buildObject"=w542) -> ()  [unwired: 3 in, 4 out]
              }
              frame "VI" {
                w577 = AB_RW_Project_PropBag_Action."writePrevious" ("action")
                w569 = AB_RW_Project_PropBag_Action."clear" ("action")
                w578 = AB_RW_Project_PropBag_Action."read" ("action")
                n190 = call <vilib>:"AB_820_850_Project_Source.vi"("action"=w578, "index in"=w583, "buildObject"=w584) -> ("index out"=w581:i32, "dataSource out"=w562:T8, "buildObject out"=w582:T1)  [unwired: 5 in, 1 out]
                n191 = Unbundle By Name(w562) -> ("itemID"=w559:string, "destinationIndex"=w567:i32)
                n192 = call <vilib>:"AB_820_850_Project_Source_VI.vi"("action"=w578, "index in"=w581, "buildObject"=w582) -> ("index out"=w580:i32, "dataSource out"=w574:T9, "buildObject out"=w579:T1)  [unwired: 5 in, 1 out]
                n193 = Unbundle By Name(w561) -> ("buildType"=w568:T2)
                n194 = call <vilib>:"AB_820_850_Project_Source.vi"("action"=w569, "index in"=w580, "buildObject"=w579) -> ("index out"=w570:i32, "buildObject out"=w572:T1)  [unwired: 5 in, 2 out]
                n195 = case shown="Default" w568 {
                  tunnel: w567 -> [w589 w591]
                  tunnel: [w589 w590] -> w565
                  frame "SourceDist" {
                  }
                  frame Default {
                    n196 = case shown="2" w591 {
                      selector: w591 -> [w592 _ _]
                      tunnel: [w592 2 ("destinationIndex") 1 ("destinationIndex")] -> w590
                      frame Default {
                      }
                      frame 1 {
                      }
                      frame 2 {
                      }
                    }
                  }
                }
                n197 = Bundle By Name(cluster=w562, "destinationIndex"=w565) -> (w563:T8)
                n198 = Search 1D Array(1D array=w560, element=w565) -> (index of element=w566:i32)  [unwired: 1 in]
                n199 = call <vilib>:"AB_820_850_Project_Source_VI.vi"("action"=w569, "index in"=w570, "buildObject"=w572) -> ("buildObject out"=w571:T1)  [unwired: 5 in, 3 out]
                n200 = case shown="Default" w566 {
                  tunnel: w565 -> [w587 _]
                  tunnel: [w586 w588] -> w564
                  tunnel: w560 -> [w585 w588]
                  frame -1 {
                    n201 = Build Array (concatenate)(w585, w587) -> (w586:i32[])
                  }
                  frame Default {
                  }
                }
                n202 = call <vilib>:"AB_820_850_Project_Source.vi"("dataForPrevious"=w561, "action"=w577, "index in"=w573, "dataSource in"=w563, "buildObject"=w571) -> ("index out"=w575:i32, "buildObject out"=w576:T1)  [unwired: 3 in, 2 out]
                n203 = call <vilib>:"AB_820_850_Project_Source_VI.vi"("dataForPrevious"=w561, "action"=w577, "index in"=w575, "dataSource in"=w574, "buildObject"=w576) -> ()  [unwired: 3 in, 4 out]
              }
              frame "ExportedVI" {
                w607 = AB_RW_Project_PropBag_Action."writePrevious" ("action")
                w603 = AB_RW_Project_PropBag_Action."clear" ("action")
                w609 = AB_RW_Project_PropBag_Action."read" ("action")
                n204 = call <vilib>:"AB_820_850_Project_Source.vi"("action"=w609, "index in"=w631, "buildObject"=w595) -> ("index out"=w629:i32, "dataSource out"=w616:T8, "buildObject out"=w630:T1)  [unwired: 5 in, 1 out]
                n205 = Unbundle By Name(w616) -> ("itemID"=w601:string, "destinationIndex"=w621:i32)
                n206 = call <vilib>:"AB_820_850_Project_Source_VI.vi"("action"=w609, "index in"=w629, "buildObject"=w630) -> ("index out"=w611:i32, "dataSource out"=w626:T9, "buildObject out"=w613:T1)  [unwired: 5 in, 1 out]
                n207 = Unbundle By Name(w615) -> ("buildType"=w622:T2)
                n208 = call <vilib>:"AB_820_850_Project_Source_ExportedVI.vi"("action"=w609, "index in"=w611, "buildObject"=w613) -> ("index out"=w610:i32, "dataSource out"=w599:cluster{"vipInfo":T10}, "buildObject out"=w612:T1)  [unwired: 5 in, 1 out]
                n209 = call <vilib>:"AB_820_850_Project_Source.vi"("action"=w603, "index in"=w610, "buildObject"=w612) -> ("index out"=w623:i32, "buildObject out"=w624:T1)  [unwired: 5 in, 2 out]
                n210 = case shown="Default" w622 {
                  tunnel: w621 -> [w636 w638]
                  tunnel: [w636 w637] -> w619
                  frame "SourceDist" {
                  }
                  frame Default {
                    n211 = case shown="2" w638 {
                      selector: w638 -> [w639 _ _]
                      tunnel: [w639 2 ("destinationIndex") 1 ("destinationIndex")] -> w637
                      frame Default {
                      }
                      frame 1 {
                      }
                      frame 2 {
                      }
                    }
                  }
                }
                n212 = call <resource>:"mxLvGetItemFromItemIDSFP.vi"("Item ID"=w601, "Item"=w595) -> ("returned Item"=w600:T1)  [unwired: 7 in, 2 out]
                n213 = call <resource>:"mxLvGetURLSFP.vi"("Item"=w600) -> ("URL"=w597:string)  [unwired: 8 in, 2 out]
                n214 = String To Path(string=w597) -> (path=w596:path)
                n215 = Bundle By Name(cluster=w616, "destinationIndex"=w619) -> (w617:T8)
                n216 = Search 1D Array(1D array=w614, element=w619) -> (index of element=w620:i32)  [unwired: 1 in]
                n217 = call <vilib>:"AB_820_850_Project_Source_VI.vi"("action"=w603, "index in"=w623, "buildObject"=w624) -> ("index out"=w604:i32, "buildObject out"=w605:T1)  [unwired: 5 in, 2 out]
                n218 = case shown="-1" w620 {
                  tunnel: w619 -> [w634 _]
                  tunnel: [w633 w635] -> w618
                  tunnel: w614 -> [w632 w635]
                  frame -1 {
                    n219 = Build Array (concatenate)(w632, w634) -> (w633:i32[])
                  }
                  frame Default {
                  }
                }
                n220 = call <vilib>:"AB_820_850_Project_Source_ExportedVI.vi"("action"=w603, "index in"=w604, "buildObject"=w605) -> ("buildObject out"=w602:T1)  [unwired: 5 in, 3 out]
                n221 = call <vilib>:"AB_820_850_Project_Source.vi"("dataForPrevious"=w615, "action"=w607, "index in"=w625, "dataSource in"=w617, "buildObject"=w602) -> ("index out"=w627:i32, "buildObject out"=w628:T1)  [unwired: 3 in, 2 out]
                n222 = call <vilib>:"AB_820_850_ConvertProtoForPrevious.vi"("Path"=w596, "dataSource in"=w599) -> ("dataSource out"=w598:cluster{"vipInfo":T10})  [unwired: 8 in, 1 out]
                n223 = call <vilib>:"AB_820_850_Project_Source_VI.vi"("dataForPrevious"=w615, "action"=w607, "index in"=w627, "dataSource in"=w626, "buildObject"=w628) -> ("index out"=w606:i32, "buildObject out"=w608:T1)  [unwired: 3 in, 2 out]
                n224 = call <vilib>:"AB_820_850_Project_Source_ExportedVI.vi"("action"=w607, "index in"=w606, "dataSource in"=w598, "buildObject"=w608) -> ()  [unwired: 4 in, 4 out]
              }
              frame "Container" {
                w662 = AB_RW_Project_PropBag_Action."writePrevious" ("action")
                w653 = AB_RW_Project_PropBag_Action."clear" ("action")
                w663 = AB_RW_Project_PropBag_Action."read" ("action")
                n225 = Bundle By Name(cluster=w644, "folder"=TRUE) -> (w656:T4)
                n226 = call <vilib>:"AB_820_850_Project_Source.vi"("action"=w663, "index in"=w668, "buildObject"=w669) -> ("index out"=w657:i32, "dataSource out"=w645:T8, "buildObject out"=w666:T1)  [unwired: 5 in, 1 out]
                n227 = Unbundle By Name(w645) -> ("itemID"=w642:string, "destinationIndex"=w650:i32)
                n228 = call <vilib>:"AB_820_850_Project_Source_Container.vi"("action"=w663, "index in"=w657, "buildObject"=w666) -> ("index out"=w660:i32, "dataSource out"=w661:T11, "buildObject out"=w665:T1)  [unwired: 5 in, 1 out]
                n229 = Unbundle By Name(w644) -> ("buildType"=w651:T2)
                n230 = call <vilib>:"AB_820_850_Project_Source.vi"("action"=w653, "index in"=w660, "buildObject"=w665) -> ("index out"=w652:i32, "buildObject out"=w655:T1)  [unwired: 5 in, 2 out]
                n231 = case shown="Default" w651 {
                  tunnel: w650 -> [w674 w676]
                  tunnel: [w674 w675] -> w648
                  frame "SourceDist" {
                  }
                  frame Default {
                    n232 = case shown="2" w676 {
                      selector: w676 -> [w677 _ _]
                      tunnel: [w677 2 ("destinationIndex") 1 ("destinationIndex")] -> w675
                      frame Default {
                      }
                      frame 1 {
                      }
                      frame 2 {
                      }
                    }
                  }
                }
                n233 = Bundle By Name(cluster=w645, "destinationIndex"=w648) -> (w646:T8)
                n234 = Search 1D Array(1D array=w643, element=w648) -> (index of element=w649:i32)  [unwired: 1 in]
                n235 = call <vilib>:"AB_820_850_Project_Source_Container.vi"("action"=w653, "index in"=w652, "buildObject"=w655) -> ("buildObject out"=w654:T1)  [unwired: 5 in, 3 out]
                n236 = case shown="Default" w649 {
                  tunnel: w648 -> [w672 _]
                  tunnel: [w671 w673] -> w647
                  tunnel: w643 -> [w670 w673]
                  frame -1 {
                    n237 = Build Array (concatenate)(w670, w672) -> (w671:i32[])
                  }
                  frame Default {
                  }
                }
                n238 = call <vilib>:"AB_820_850_Project_Source.vi"("dataForPrevious"=w656, "action"=w662, "index in"=w667, "dataSource in"=w646, "buildObject"=w654) -> ("index out"=w659:i32, "buildObject out"=w664:T1)  [unwired: 3 in, 2 out]
                n239 = call <vilib>:"AB_820_850_Project_Source_Container.vi"("action"=w662, "index in"=w659, "dataSource in"=w661, "buildObject"=w664) -> ()  [unwired: 4 in, 4 out]
              }
              frame "Library" {
                w680 = TRUE ("folder")
                w702 = AB_RW_Project_PropBag_Action."writePrevious" ("action")
                w699 = AB_RW_Project_PropBag_Action."clear" ("action")
                w701 = AB_RW_Project_PropBag_Action."read" ("action")
                n240 = Bundle By Name(cluster=w691, "folder"=w680, "isLibrary"=w680) -> (w697:T4)
                n241 = call <vilib>:"AB_820_850_Project_Source.vi"("action"=w701, "index in"=w706, "buildObject"=w707) -> ("index out"=w686:i32, "dataSource out"=w690:T8, "buildObject out"=w687:T1)  [unwired: 5 in, 1 out]
                n242 = Unbundle By Name(w690) -> ("itemID"=w681:string, "destinationIndex"=w695:i32)
                n243 = Unbundle By Name(w691) -> ("buildType"=w696:T2)
                n244 = call <vilib>:"AB_820_850_Project_Source_Library.vi"("action"=w701, "index in"=w686, "buildObject"=w687) -> ("index out"=w703:i32, "dataSource out"=w700:T12, "buildObject out"=w704:T1)  [unwired: 5 in, 1 out]
                n245 = call <vilib>:"AB_820_850_Project_Source.vi"("action"=w699, "index in"=w703, "buildObject"=w704) -> ("index out"=w685:i32, "buildObject out"=w684:T1)  [unwired: 5 in, 2 out]
                n246 = case shown="Default" w696 {
                  tunnel: w695 -> [w712 w714]
                  tunnel: [w712 w713] -> w693
                  frame "SourceDist" {
                  }
                  frame Default {
                    n247 = case shown="Default" w714 {
                      selector: w714 -> [w715 _ _]
                      tunnel: [w715 2 ("destinationIndex") 1 ("destinationIndex")] -> w713
                      frame Default {
                      }
                      frame 1 {
                      }
                      frame 2 {
                      }
                    }
                  }
                }
                n248 = Bundle By Name(cluster=w690, "destinationIndex"=w693) -> (w689:T8)
                n249 = Search 1D Array(1D array=w688, element=w693) -> (index of element=w694:i32)  [unwired: 1 in]
                n250 = call <vilib>:"AB_820_850_Project_Source_Library.vi"("action"=w699, "index in"=w685, "buildObject"=w684) -> ("buildObject out"=w698:T1)  [unwired: 5 in, 3 out]
                n251 = case shown="-1" w694 {
                  tunnel: w693 -> [w710 _]
                  tunnel: [w709 w711] -> w692
                  tunnel: w688 -> [w708 w711]
                  frame -1 {
                    n252 = Build Array (concatenate)(w708, w710) -> (w709:i32[])
                  }
                  frame Default {
                  }
                }
                n253 = call <vilib>:"AB_820_850_Project_Source.vi"("dataForPrevious"=w697, "action"=w702, "index in"=w705, "dataSource in"=w689, "buildObject"=w698) -> ("index out"=w682:i32, "buildObject out"=w683:T1)  [unwired: 3 in, 2 out]
                n254 = call <vilib>:"AB_820_850_Project_Source_Library.vi"("action"=w702, "index in"=w682, "dataSource in"=w700, "buildObject"=w683) -> ()  [unwired: 4 in, 4 out]
              }
            }
            n255 = Build Array (concatenate)(w514, w516) -> (w515:string[])
          }
          n256 = case shown="\"SourceDist\"" w452 {
            tunnel: w453 -> [_ w494]
            tunnel: w451 -> [_ w487]
            tunnel: T8 {"itemID"="", "sourceInclusion"=enum."IncludeIfReferenced", "destinationIndex"=0, "properties"=[], "newName"="", "lvfile"=FALSE} ("dataSource in") -> [_ w492]
            tunnel: w449 -> [_ w491]
            tunnel: w448 -> [_ w490]
            tunnel: w447 -> [_ w486]
            frame Default {
            }
            frame "SourceDist" {
              # "Remove dependency node"
              n257 = call <resource>:"mxLvGetAllDescendentsSFP.vi"("Provider Item"=w486, "Item"=w487) -> ("Descendents"=w485:T1[])  [unwired: 7 in, 2 out]
              n258 = Array Size(array=w494) -> (size(s)=w493:i32)
              n259 = Decrement(x=w493) -> (x-1=w488:i32)
              n260 = for {
                tunnel: w485 -> [w496] mode=indexing
                tunnel: w494 -> [w503]
                shift-right: [w499] -> w489
                shift-left: w488 -> [w500]
                tunnel: w487 -> [w502]
                tunnel: w492 -> [w498]
                tunnel: w491 -> [w497]
                n261 = call <resource>:"mxLvGetItemIDFromItemSFP.vi"("Item"=w496) -> ("Item ID"=w495:string)  [unwired: 8 in, 2 out]
                n262 = Search 1D Array(1D array=w503, element=w495) -> (index of element=w501:i32)  [unwired: 1 in]
                n263 = case shown="-1" w501 {
                  tunnel: w502 -> [_ w513]
                  tunnel: w500 -> [w504 w512]
                  tunnel: [w504 w511] -> w499
                  tunnel: w498 -> [_ w510]
                  tunnel: w495 -> [_ w509]
                  tunnel: w497 -> [_ w506]
                  frame Default {
                  }
                  frame -1 {
                    n264 = Bundle By Name(cluster=w510, "itemID"=w509, "sourceInclusion"=AB_Source_Inclusion."IncludeIfReferenced") -> (w507:T8)
                    n265 = call <vilib>:"AB_820_850_Project_Source.vi"("dataForPrevious"=w506, "action"=AB_RW_Project_PropBag_Action."writePrevious", "index in"=w512, "dataSource in"=w507, "buildObject"=w513) -> ()  [unwired: 3 in, 4 out]
                    n266 = Increment(x=w512) -> (x+1=w511:i32)
                  }
                }
              }
              n267 = call <resource>:"mxLvSetIntProperty.vi"("Value (0)"=w489, "Tag"=w490, "Item"=w487) -> ()  [unwired: 7 in, 2 out]
            }
          }
        }
        frame "clear" {
          n268 = call <resource>:"mxLvGetIntProperty.vi"("Tag"=w718, "Item"=w723) -> ("Value"=w721:i32, "Item"=w720:T1)  [unwired: 7 in, 1 out]
          n269 = call <resource>:"mxLvDeleteProperty.vi"("Tag"=w718, "Item"=w720) -> ("Item"=w719:T1)  [unwired: 8 in, 1 out]
          n270 = for {
            N: w721 -> [_]
            tunnel: w722 -> [w730]
            tunnel: w719 -> [w727]
            i -> [w729]
            n271 = Format Into String(format string=w730, w729) -> (resulting string=w725:string)  [unwired: 2 in, 1 out]
            n272 = call <resource>:"mxLvGetStringProperty.vi"("Tag"=w725, "Item"=w727) -> ("Value"=w724:string, "Item"=w728:T1)  [unwired: 7 in, 1 out]
            n273 = call <resource>:"mxLvDeleteProperty.vi"("Tag"=w725, "Item"=w728) -> ("Item"=w726:T1)  [unwired: 8 in, 1 out]
            n274 = case shown="\"\", \"Source\"" w724 {
              tunnel: w726 -> [_ w733 w738 w745 w750 w757]
              tunnel: w729 -> [_ w732 w737 w744 w749 w756]
              frame Default {
              }
              frame "", "Source" {
                # "For 8.5 and greater, \"Source\" class type is not written to the property bags. So if the type is an empty string, we assume it is a source type. \nWhen we load from previous, the \"Source\" tag is written to the property bag, so we need to keep the string for that reason."
                n275 = call <vilib>:"AB_820_850_Project_Source.vi"("action"=AB_RW_Project_PropBag_Action."clear", "index in"=w732, "buildObject"=w733) -> ()  [unwired: 5 in, 4 out]
              }
              frame "VI" {
                w734 = AB_RW_Project_PropBag_Action."clear" ("action")
                n276 = call <vilib>:"AB_820_850_Project_Source.vi"("action"=w734, "index in"=w737, "buildObject"=w738) -> ("index out"=w735:i32, "buildObject out"=w736:T1)  [unwired: 5 in, 2 out]
                n277 = call <vilib>:"AB_820_850_Project_Source_VI.vi"("action"=w734, "index in"=w735, "buildObject"=w736) -> ()  [unwired: 5 in, 4 out]
              }
              frame "ExportedVI" {
                w741 = AB_RW_Project_PropBag_Action."clear" ("action")
                n278 = call <vilib>:"AB_820_850_Project_Source.vi"("action"=w741, "index in"=w744, "buildObject"=w745) -> ("index out"=w742:i32, "buildObject out"=w743:T1)  [unwired: 5 in, 2 out]
                n279 = call <vilib>:"AB_820_850_Project_Source_VI.vi"("action"=w741, "index in"=w742, "buildObject"=w743) -> ("index out"=w739:i32, "buildObject out"=w740:T1)  [unwired: 5 in, 2 out]
                n280 = call <vilib>:"AB_820_850_Project_Source_ExportedVI.vi"("action"=w741, "index in"=w739, "buildObject"=w740) -> ()  [unwired: 5 in, 4 out]
              }
              frame "Container" {
                w747 = AB_RW_Project_PropBag_Action."clear" ("action")
                n281 = call <vilib>:"AB_820_850_Project_Source.vi"("action"=w747, "index in"=w749, "buildObject"=w750) -> ("index out"=w746:i32, "buildObject out"=w748:T1)  [unwired: 5 in, 2 out]
                n282 = call <vilib>:"AB_820_850_Project_Source_Container.vi"("action"=w747, "index in"=w746, "buildObject"=w748) -> ()  [unwired: 5 in, 4 out]
              }
              frame "Library" {
                w752 = AB_RW_Project_PropBag_Action."clear" ("action")
                n283 = call <vilib>:"AB_820_850_Project_Source.vi"("action"=w752, "index in"=w756, "buildObject"=w757) -> ("index out"=w754:i32, "buildObject out"=w755:T1)  [unwired: 5 in, 2 out]
                n284 = call <vilib>:"AB_820_850_Project_Source_Container.vi"("action"=w752, "index in"=w754, "buildObject"=w755) -> ("index out"=w751:i32, "buildObject out"=w753:T1)  [unwired: 5 in, 2 out]
                n285 = call <vilib>:"AB_820_850_Project_Source_Library.vi"("action"=w752, "index in"=w751, "buildObject"=w753) -> ()  [unwired: 5 in, 4 out]
              }
            }
          }
        }
      }
    }
    frame Error {
    }
  }
  "usedDestinations" <- w3
  "error out" <- "error in (no error)"
  "buildObject out" <- "buildObject"
